vi "SW Interface - SET -  Actor_Name.vi"(8 "error in (no error)":errorcluster, 10 "Actor_Name":string, 11 "SW_Interface_Actor.lvlib:SW_Interface_Class.lvclass":refnum<class "SW_Interface_Class.lvclass">) -> (0 "error out":errorcluster, 2 "Actor Name":string, 3 "SW_Interface_Actor.lvlib:SW_Interface_Class.lvclass 2":refnum<class "SW_Interface_Class.lvclass">)   [LabVIEW 2023, in "SW_Interface_Actor.lvlib" / "SW_Interface_Class.lvclass"]
uses:
  SW_Interface_Class.lvclass
  <vilib>/Utility/error.llb/Trim Whitespace One-Sided.vi
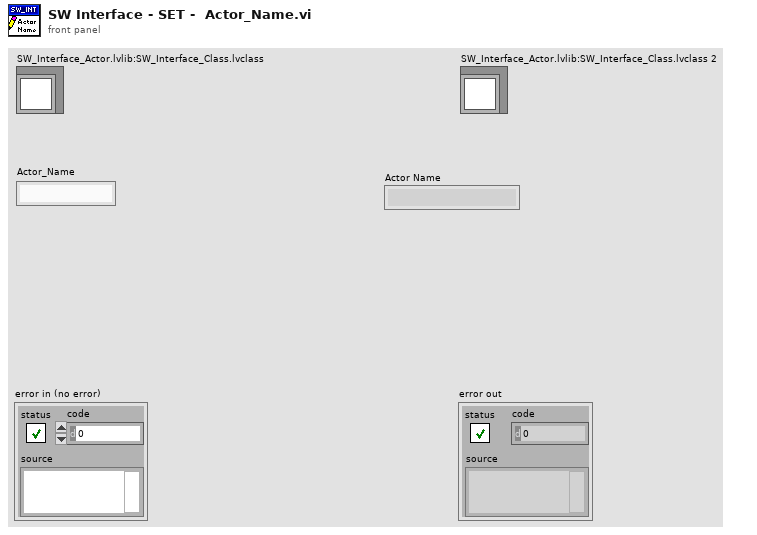
[diagram p1: front panel]
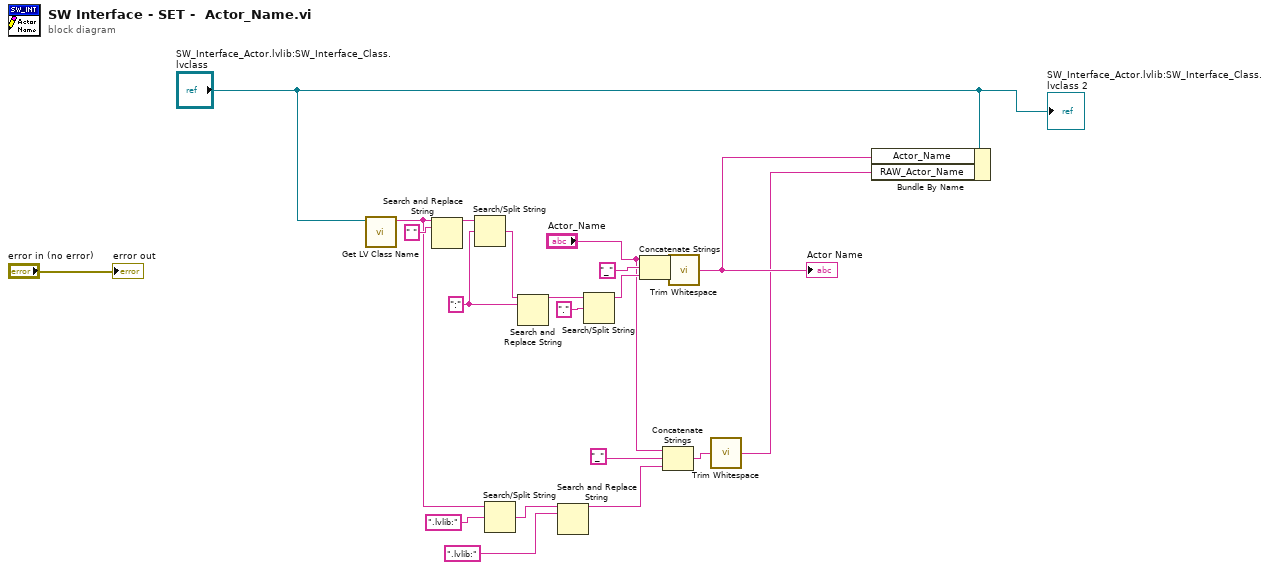
[diagram p0: block diagram]
diagram:
  w18 = ":" ("search string/char (-)")
  n1 = call <vilib>:"Get LV Class Name.vi"("object"="SW_Interface_Actor.lvlib:SW_Interface_Class.lvclass") -> ("class name"=w7:string)  [unwired: 9 in, 1 out]
  n2 = Search and Replace String(input string=w7, search string=" ") -> (result string=w20:string)  [unwired: 6 in, 3 out]
  n3 = Search/Split String(string=w20, search string/char (-)=w18) -> (match + rest of string=w19:string)  [unwired: 1 in, 2 out]
  n4 = Search/Split String(string=w7, search string/char (-)=".lvlib:") -> (match + rest of string=w10:string)  [unwired: 1 in, 2 out]
  n5 = Search and Replace String(input string=w19, search string=w18) -> (result string=w15:string)  [unwired: 6 in, 3 out]
  n6 = Search and Replace String(input string=w10, search string=".lvlib:" ("search string/char (-)")) -> (result string=w9:string)  [unwired: 6 in, 3 out]
  n7 = Search/Split String(string=w15, search string/char (-)=".") -> (substring before match=w13:string)  [unwired: 1 in, 2 out]
  n8 = Concatenate Strings("Actor_Name", "_" ("string"), w13) -> (w16:string)
  n9 = Concatenate Strings("Actor_Name", "_" ("string"), w9) -> (w8:string)
  n10 = call <vilib>:"Trim Whitespace.vi"("string"=w16) -> ("trimmed string"=w2:string)  [unwired: 1 in]
  "Actor Name" <- w2
  n11 = call <vilib>:"Trim Whitespace.vi"("string"=w8) -> ("trimmed string"=w1:string)  [unwired: 1 in]
  n12 = Bundle By Name(cluster="SW_Interface_Actor.lvlib:SW_Interface_Class.lvclass", "Actor_Name"=w2, "RAW_Actor_Name"=w1) -> ()  [unwired: 1 out]
  "error out" <- "error in (no error)"
  "SW_Interface_Actor.lvlib:SW_Interface_Class.lvclass 2" <- "SW_Interface_Actor.lvlib:SW_Interface_Class.lvclass"
